vi "Begin.vi"(10 "error in (no error)":errorcluster, 11 "FPGA VI Reference In":T1) -> (2 "error out":errorcluster, 3 "FPGA VI Reference Out":T1)   [LabVIEW 2016]
uses:
  FPGA Bitfiles/FPGA_defref.ctl
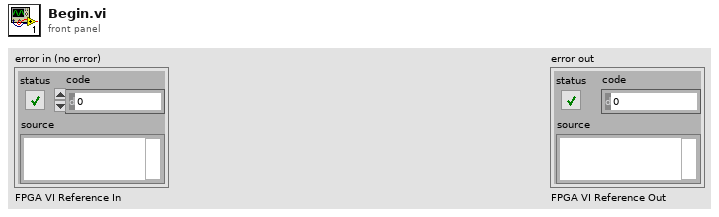
[diagram p1: front panel]
types:
  T1 = typedef "FPGA_defref.ctl" = refnum<k20>
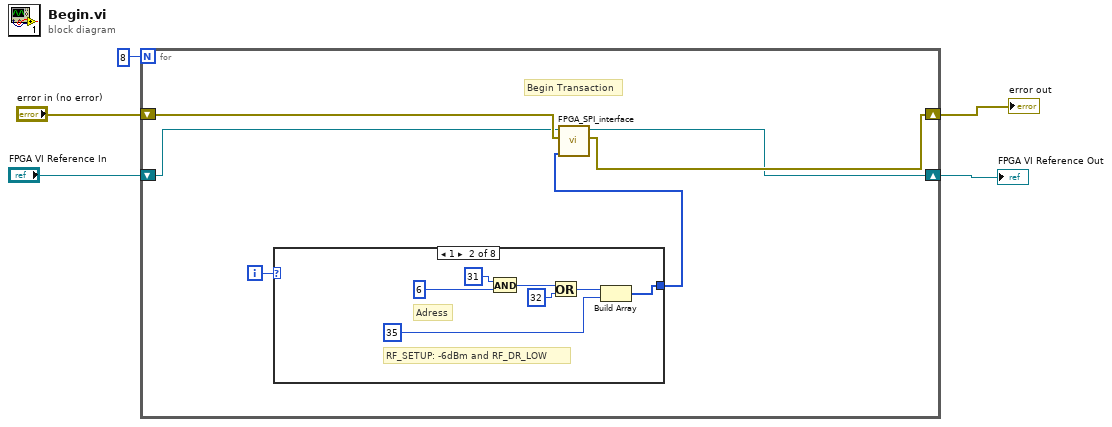
[diagram p0: block diagram]
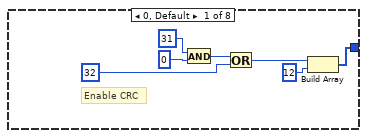
[diagram p2: hidden frame]
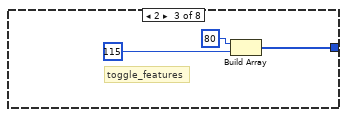
[diagram p3: hidden frame]
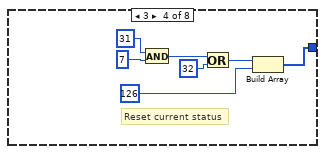
[diagram p4: hidden frame]
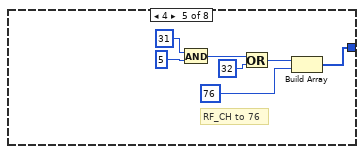
[diagram p5: hidden frame]
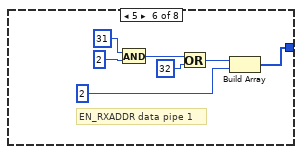
[diagram p6: hidden frame]
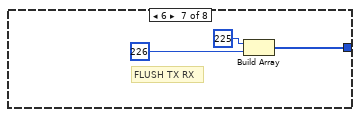
[diagram p7: hidden frame]
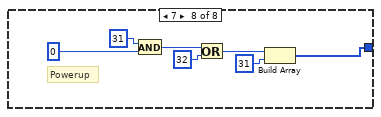
[diagram p8: hidden frame]
diagram:
  n1 = for {
    N: 8 -> [_]
    shift-right: [w9] -> w3
    shift-left: "error in (no error)" -> [w8]
    shift-right: [w7] -> w2
    shift-left: "FPGA VI Reference In" -> [w6]
    i -> [w11]
    # "Begin Transaction"
    n2 = case shown="1" w11 {
      tunnel: [w12 w19 w26 w29 w37 w43 w50 w53] -> w10
      frame 0, Default {
        # "Enable CRC"
        n3 = And(x=31, y=0) -> (x .and. y?=w16:i32)
        n4 = Or(x=w16, y=32) -> (x .or. y?=w18:i32)
        n5 = Build Array(w18, 12) -> (w12:i32[])
      }
      frame 1 {
        # "RF_SETUP: -6dBm and RF_DR_LOW"
        # "Adress"
        n6 = And(x=31, y=6) -> (x .and. y?=w23:i32)
        n7 = Or(x=w23, y=32) -> (x .or. y?=w25:i32)
        n8 = Build Array(w25, 35) -> (w19:i32[])
      }
      frame 2 {
        # "toggle_features"
        n9 = Build Array(80, 115) -> (w26:i32[])
      }
      frame 3 {
        # "Reset current status"
        n10 = And(x=31, y=7) -> (x .and. y?=w33:i32)
        n11 = Or(x=w33, y=32) -> (x .or. y?=w35:i32)
        n12 = Build Array(w35, 126) -> (w29:i32[])
      }
      frame 4 {
        # "RF_CH to 76"
        n13 = And(x=31, y=5) -> (x .and. y?=w40:i32)
        n14 = Or(x=w40, y=32) -> (x .or. y?=w42:i32)
        n15 = Build Array(w42, 76) -> (w37:i32[])
      }
      frame 5 {
        # "EN_RXADDR data pipe 1"
        n16 = And(x=31, y=2) -> (x .and. y?=w47:i32)
        n17 = Or(x=w47, y=32) -> (x .or. y?=w49:i32)
        n18 = Build Array(w49, 2) -> (w43:i32[])
      }
      frame 6 {
        # "FLUSH TX RX"
        n19 = Build Array(225, 226) -> (w50:i32[])
      }
      frame 7 {
        # "Powerup"
        n20 = And(x=31, y=0) -> (x .and. y?=w57:i32)
        n21 = Or(x=w57, y=32) -> (x .or. y?=w59:i32)
        n22 = Build Array(w59, 31) -> (w53:i32[])
      }
    }
    n23 = call "FPGA_SPI_interface.vi"("Frames to Write"=w10, "error in"=w8, "FPGA VI Reference In"=w6) -> ("error out"=w9:errorcluster, "FPGA VI Reference Out"=w7:T1)  [unwired: 6 in, 1 out]
  }
  "error out" <- w3
  "FPGA VI Reference Out" <- w2
